vi "SubVI_Example_LabVIEW_Enable_Control.vi"(11 "UI Control (Reference)":refnum<vi>) -> ()   [LabVIEW 2010]
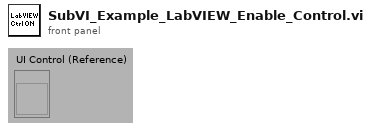
[diagram p1: front panel]
types:
  T1 = enum8{"Enabled", "Disabled", "Disabled and Grayed Out"}
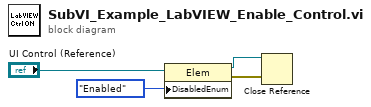
[diagram p0: block diagram]
diagram:
  n1 = property class="Elem"(reference="UI Control (Reference)", "DisabledEnum"=T1."Enabled" ("Disabled")) -> (reference out=w1:refnum<vi>, error out=w2:errorcluster)  [unwired: 1 in]
  n2 = Close Reference ("Close Referenz")(reference=w1, error in (no error)=w2) -> ()  [unwired: 1 out]
